vi "TEST_bench_fgm_partial_pipeline.vi"() -> ()   [LabVIEW 2017]
uses:
  fixed-point/single-axis/fxp_mpc/fgm_pipiline/quadProgParams_pipe.ctl
  <vilib>/rvi/Emulation/niFpgaEmulationIsFPGAContextNoSignature.vi
  <vilib>/rvi/DataTransferAndStorage/Container/Common/niFpgaContainerGetUniqueNameForEmu.vi
  <vilib>/rvi/Memory/Memory_Emulation/niFpgaMemoryEmulationCacheClearOnFirstRun.vi
  <vilib>/rvi/Memory/Memory_Emulation/nirvimemoryEmulationManagerCache_MakeExclusive.vi
  <vilib>/rvi/Memory/Memory_Emulation/niFpgaMemoryEmulationValidateCache.vi
  <vilib>/rvi/Memory/Memory_Emulation/nirvimemoryEmulationManagerCache_InsertValue.vi
  <vilib>/Utility/error.llb/Clear Errors.vi
  <vilib>/rvi/Memory/Memory_Emulation/nirvimemoryEmulationManagerCache_ReleaseExclusive.vi
  <vilib>/rvi/Memory/Memory_Emulation/nirvimemoryEmulationManagerCache_GetValue.vi
  <vilib>/rvi/Memory/Memory_Emulation/nirvimemoryEmulationManagerCache_SetValue.vi
  <vilib>/rvi/Emulation/niFpgaProcessEmulError.vi
  <vilib>/rvi/Emulation/niFpgaSctlEmulationGetInTimedLoop.vi
  <vilib>/rvi/Memory/Memory_Emulation/nirvimemoryFastEmulation.vi
  <vilib>/rvi/Memory/Memory_Emulation/nirvimemoryEmulation.vi
  <vilib>/rvi/errors/nirviReportUnexpectedCaseInternalError (U32).vi
  <vilib>/rvi/DataTransferAndStorage/Container/XNode/niFpgaContainer.xnode
  <vilib>/rvi/DataTransferAndStorage/Register/Emulation/niFpgaRegisterEmulation.vi
panel:
  in  "du_max":fxp<+/-,18,1>
  in  "QP_params":T1={"maxIter"=0, "nuN"=24, "Ns_mpc"=0, "-beta"=-0.9987945556640625, "beta+1"=1.9987945556640625}
  in  "idx2":i16=15
  in  "idx1":i16
  out "idx1":fxp<+/-,32,6>[](array[numeric])
  out "idx2":fxp<+/-,32,6>[](array[numeric])
  in  "z0":fxp<+/-,32,6>[](array[numeric])=[0.0, 0.0, 0.0, 0.0, 0.0, 0.0, 0.0, 0.0, 0.0, 0.0, 0.0, 0.0]
  in  "y0":fxp<+/-,32,6>[](array[numeric])=[0.0, 0.0, 0.0, 0.0, 0.0, 0.0, 0.0, 0.0, 0.0, 0.0, 0.0, 0.0]
  out "y":fxp<+/-,32,6>[](array[numeric])
  out "z":fxp<+/-,32,6>[](array[numeric])
  out "delta u(k)":fxp<+/-,32,3>
  in  "big_mat_data":fxp<+/-,32,3>[](array[numeric])=[0.0, 0.0, 0.0, 0.0, 0.0, 0.0, 0.0, 0.0, 0.0, 0.0, 0.0, 0.0]
  in  "x":fxp<+/-,32,6>[](array[numeric])=[0.0, 0.0, 0.0, 0.0, 0.0, 0.0, 0.0, 0.0, 0.0, 0.0, 0.0, 0.0, 0.0, 0.0, 0.0, 0.0, 0.0, 0.0, 0.0, 0.0, 0.0, 0.0, 0.0, 0.0, 0.0]
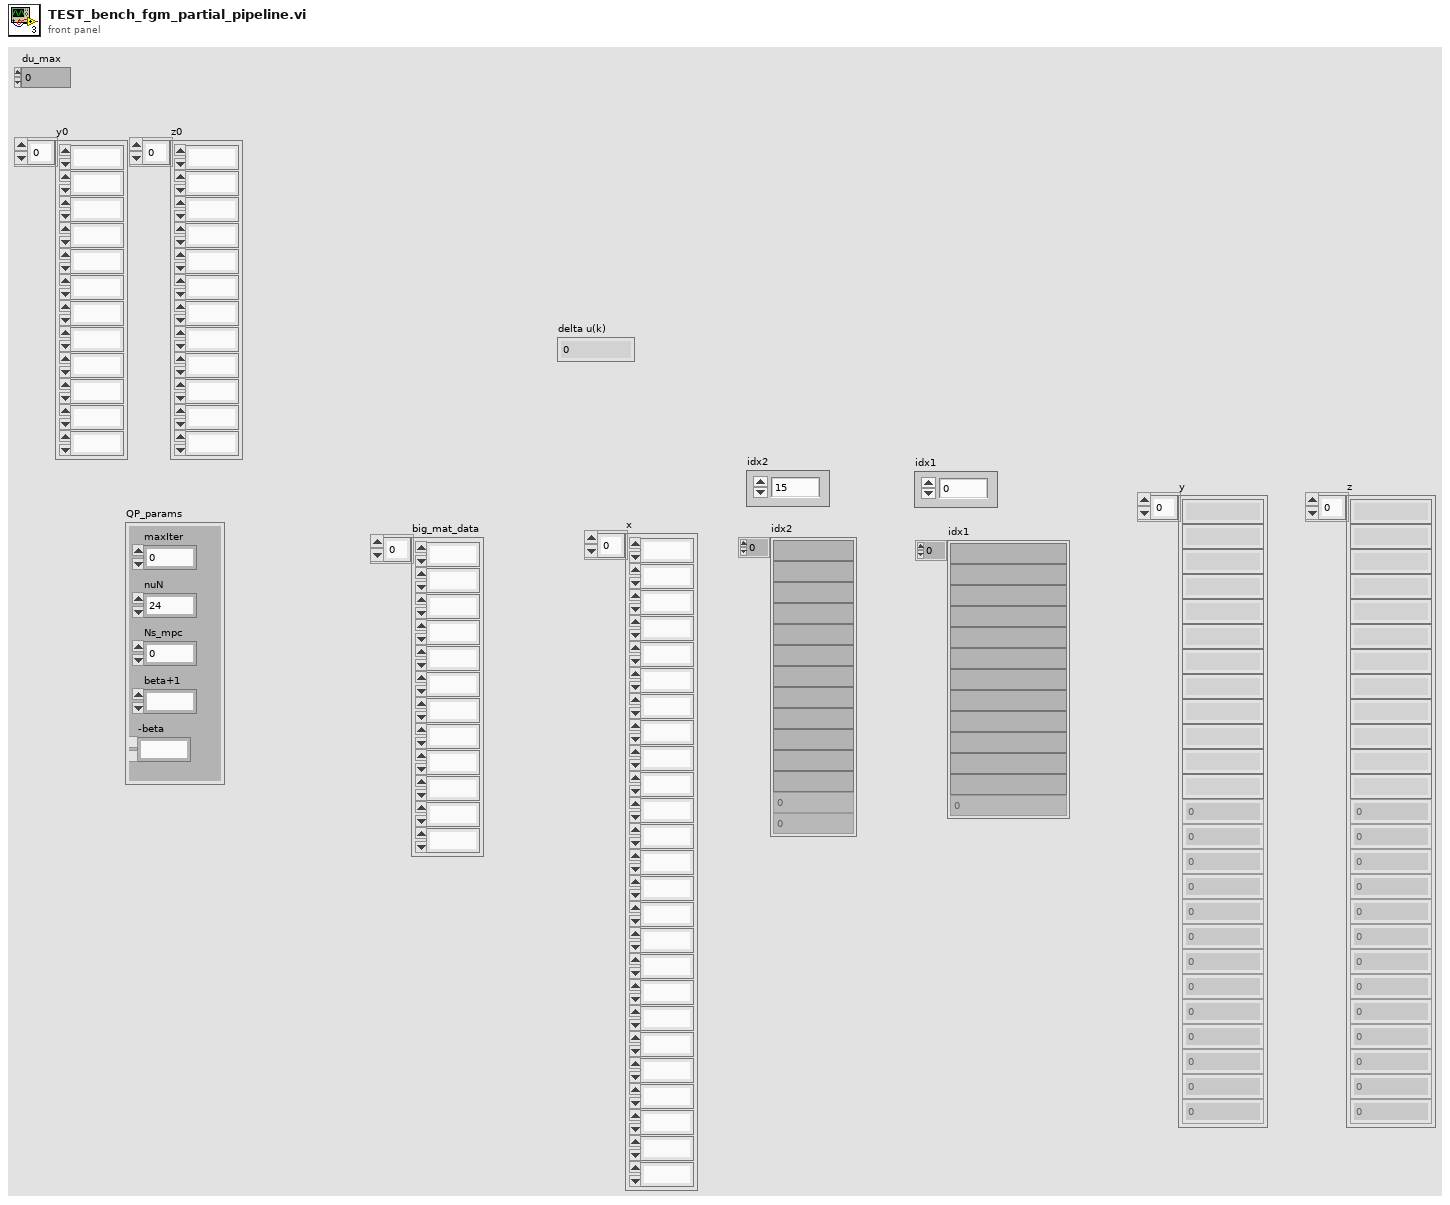
[diagram p1: front panel]
types:
  T1 = typedef "quadProgParams_pipe.ctl" = cluster{"maxIter":u16, "nuN":u16, "Ns_mpc":u16, "-beta":fxp<+/-,18,2>, "beta+1":fxp<+/-,18,2>}
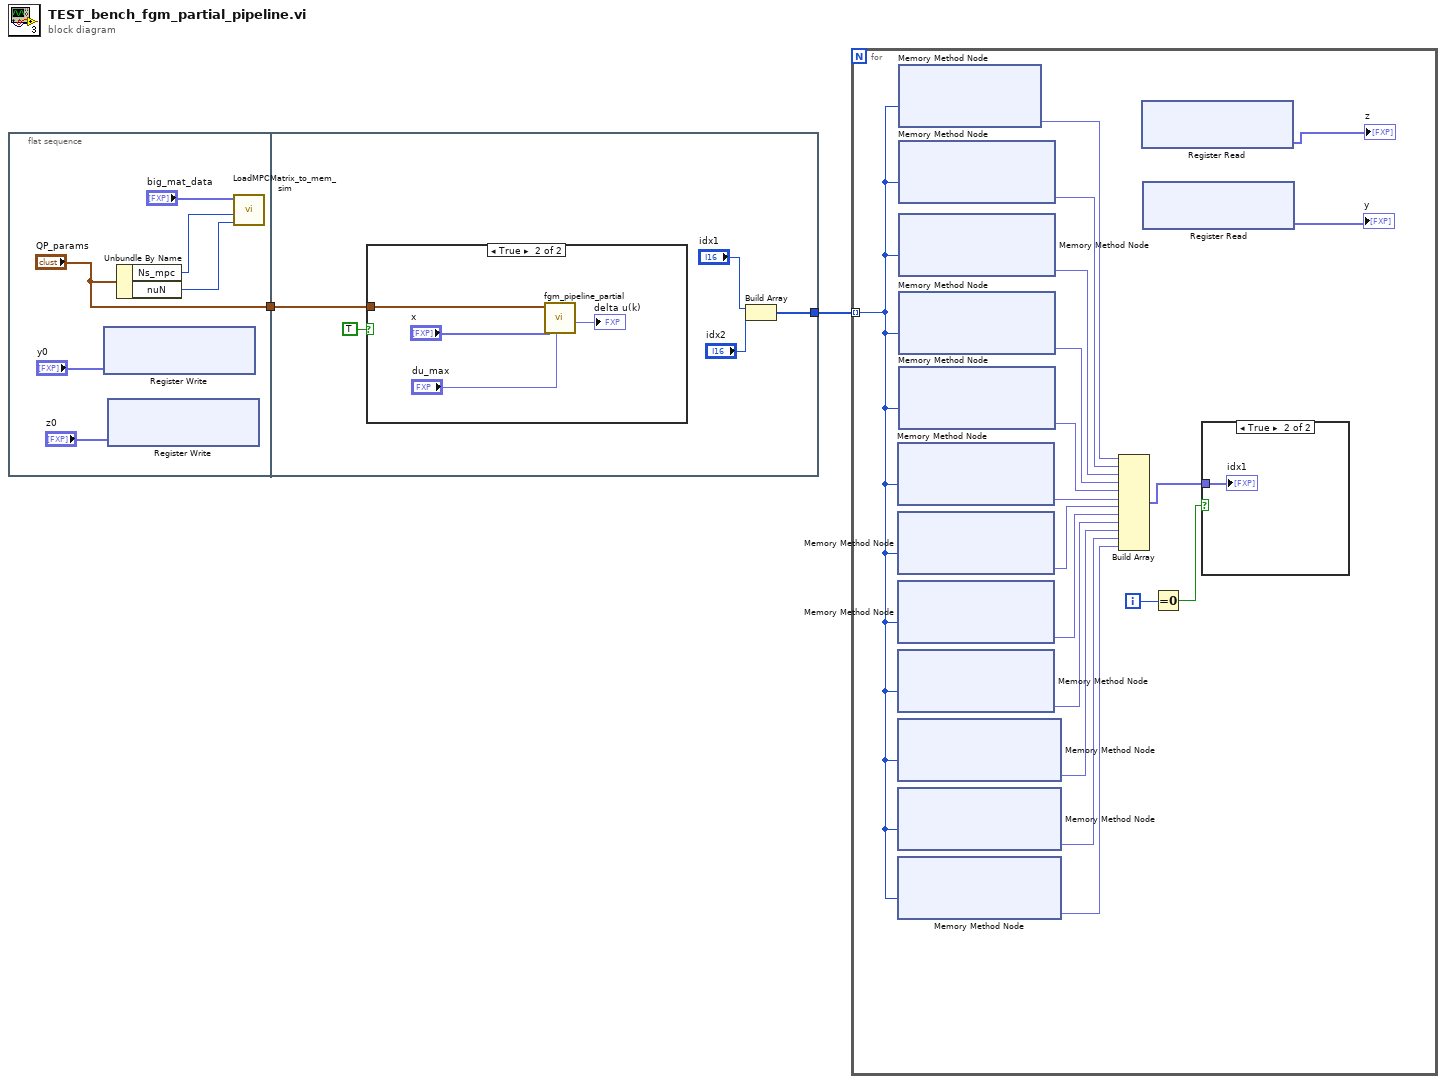
[diagram p0: block diagram]
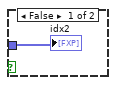
[diagram p3: hidden frame]
diagram:
  n1 = flat-sequence {
    tunnel: ["QP_params"] -> w1
    tunnel: [w13] -> w2
    tunnel: w1 -> [w12]
    frame #0 {
      n2 = xnode "Register Write"("Data"="y0") -> ()  [unwired: 1 in, 1 out]
      n3 = xnode "Register Write"("Data"="z0") -> ()  [unwired: 1 in, 1 out]
      n4 = Unbundle By Name("QP_params") -> ("Ns_mpc"=w6:u16, "nuN"=w7:u16)
      n5 = call "LoadMPCMatrix_to_mem_sim.vi"("nuN_mpc"=w7, "Ns"=w6, "big_mat_data"="big_mat_data") -> ()  [unwired: 9 in]
    }
    frame #1 {
      n6 = case shown="True" TRUE {
        tunnel: w12 -> [_ w15]
        frame False {
        }
        frame True {
          n7 = call "fgm_pipeline_partial.vi"("du_max"="du_max", "x_vec"="x", "QP_params"=w15) -> ("delta u(k)"=→"delta u(k)":fxp<+/-,32,3>)  [unwired: 6 in, 2 out]
        }
      }
      n8 = Build Array("idx1", "idx2") -> (w13:i16[])
    }
  }
  n9 = for {
    tunnel: w2 -> [w35] mode=indexing
    i -> [w20]
    n10 = xnode ("Memory Method Node")("Address"=w35) -> ("Data"=w29:fxp<+/-,32,3>)  [unwired: 1 in, 1 out]
    n11 = xnode ("Memory Method Node")("Address"=w35) -> ("Data"=w28:fxp<+/-,32,3>)  [unwired: 1 in, 1 out]
    n12 = xnode ("Memory Method Node")("Address"=w35) -> ("Data"=w27:fxp<+/-,32,3>)  [unwired: 1 in, 1 out]
    n13 = xnode ("Memory Method Node")("Address"=w35) -> ("Data"=w26:fxp<+/-,32,3>)  [unwired: 1 in, 1 out]
    n14 = xnode ("Memory Method Node")("Address"=w35) -> ("Data"=w25:fxp<+/-,32,3>)  [unwired: 1 in, 1 out]
    n15 = xnode ("Memory Method Node")("Address"=w35) -> ("Data"=w24:fxp<+/-,32,3>)  [unwired: 1 in, 1 out]
    n16 = xnode ("Memory Method Node")("Address"=w35) -> ("Data"=w23:fxp<+/-,32,3>)  [unwired: 1 in, 1 out]
    n17 = xnode ("Memory Method Node")("Address"=w35) -> ("Data"=w34:fxp<+/-,32,3>)  [unwired: 1 in, 1 out]
    n18 = xnode ("Memory Method Node")("Address"=w35) -> ("Data"=w33:fxp<+/-,32,3>)  [unwired: 1 in, 1 out]
    n19 = xnode ("Memory Method Node")("Address"=w35) -> ("Data"=w32:fxp<+/-,32,3>)  [unwired: 1 in, 1 out]
    n20 = xnode ("Memory Method Node")("Address"=w35) -> ("Data"=w31:fxp<+/-,32,3>)  [unwired: 1 in, 1 out]
    n21 = xnode ("Memory Method Node")("Address"=w35) -> ("Data"=w30:fxp<+/-,32,3>)  [unwired: 1 in, 1 out]
    n22 = Build Array(w34, w33, w32, w31, w30, w29, w28, w27, w26, w25, w24, w23) -> (w21:fxp<+/-,32,3>[])
    n23 = xnode "Register Read"() -> ("Data"=→"z":fxp<+/-,32,6>[])  [unwired: 1 in, 1 out]
    n24 = xnode "Register Read"() -> ("Data"=→"y":fxp<+/-,32,6>[])  [unwired: 1 in, 1 out]
    n25 = Equal To 0?(x=w20) -> (x = 0?=w22:bool)
    n26 = case shown="True" w22 {
      tunnel: w21 -> [w36 w37]
      frame False {
        "idx2" <- w36
      }
      frame True {
        "idx1" <- w37
      }
    }
  }
